vi "Settings - NI 9234.vi"(8 "Error In":errorcluster) -> (0 "Error Out":errorcluster={"status"=TRUE, "code"=-200077, "source"="Property Node DAQmx Channel (arg 2) in DAQmx Create Channel (AI-Temperature-Thermocouple).vi:1->Settings - NI 9211.vi <append>\n<B>Property: </B>AI.Temp.Units\n<B>Requested Value: </B>\n<B>You Can Select: </B>Deg C, Deg F, Kelvins, Deg R, From Custom Scale\n\n<B>Channel Name: </B>Temperature\n\n<B>Task Name: </B>_unnamedTask<E>"}, 3 "Cancelled?":bool)   [LabVIEW 2011]
doc: "This VI will get settings for NI 9211 measurement."
uses:
  SubVIs/Controls/4ch.ctl
  SubVIs/Controls/TransparencyEffectOperations.ctl
  <vilib>/DAQmx/create/channels.llb/DAQmx Create Channel (AI-Acceleration-Accelerometer).vi
  <vilib>/DAQmx/configure/timing.llb/DAQmx Timing (Sample Clock).vi
  Program Files/National Instruments/LabVIEW 2011/resource/objmgr/daqmx.rc
panel:
  in  "Rate":dbl=25600.0
  in  "Nr of Samples":i32=10000
  in  "Sample Mode":i32(ring)=10123 items=["Finite Samples"=10178, "Continuous Samples"=10123, "Hardware Timed Single Point"=12522]
  in  "dB Reference":dbl=1.0
  in  "Sensitivity":dbl=1000.0
  in  "Sensitivity Units":i32(ring)=12509 items=["mVolts/g"=12509, "Volts/g"=12510]
  in  "Unit":i32(ring)=10186 items=["g"=10186, "m/s^2"=12470, "From Custom Scale"=10065]
  in  "Input Terminal Configuration":i32(ring)=12529 items=["default"=-1, "RSE"=10083, "NRSE"=10078, "Differential"=10106, "Pseudodifferential"=12529]
  in  "Excitation Source":i32(ring)=10200 items=["Internal"=10200, "External"=10167, "None"=10230]
  in  "Excitation Value":dbl=0.002
  in  "Channel":T1
  in  "Min":dbl=-5.0
  in  "Max":dbl=5.0
  in  "Header For Measurement File":string="Acceleration 1"
  in  "Cancel Button":bool
  in  "OK Button":bool
  # "NI 9234"
  # "Meas File Settings"
  # "Hardware Settings"
  # "Signal Input Range"
  # "Units"
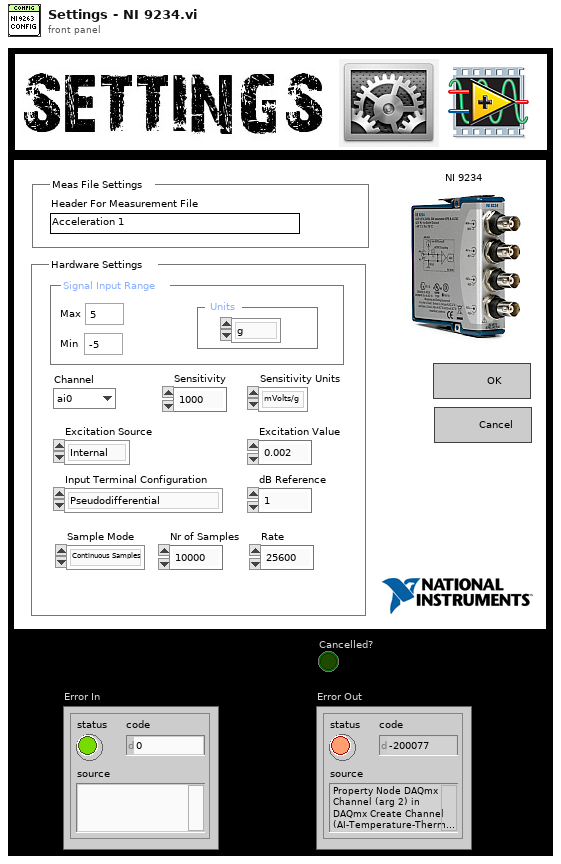
[diagram p1: front panel]
types:
  T1 = typedef "4ch.ctl" = enum16{"ai0", "ai1", "ai2", "ai3"}
  T2 = typedef "TransparencyEffectOperations.ctl" = enum16{"Show", "Hide 80%", "Hide All"}
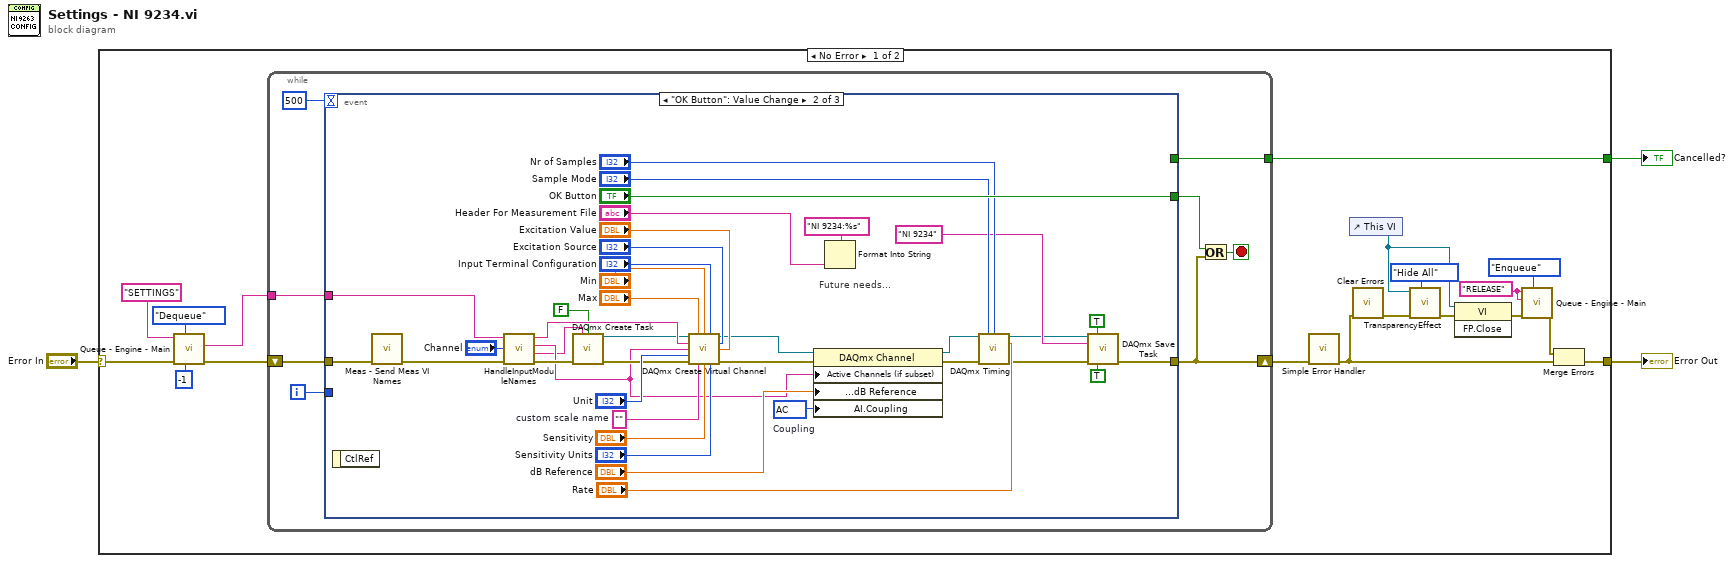
[diagram p0: block diagram]
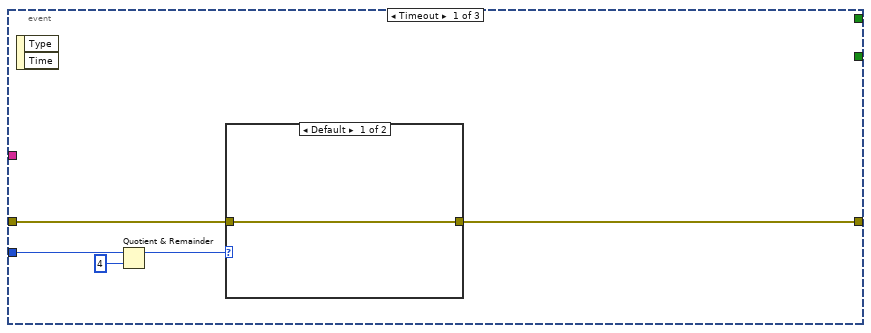
[diagram p2: hidden frame]
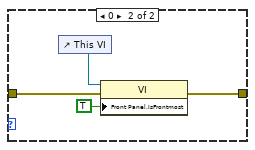
[diagram p3: hidden frame]
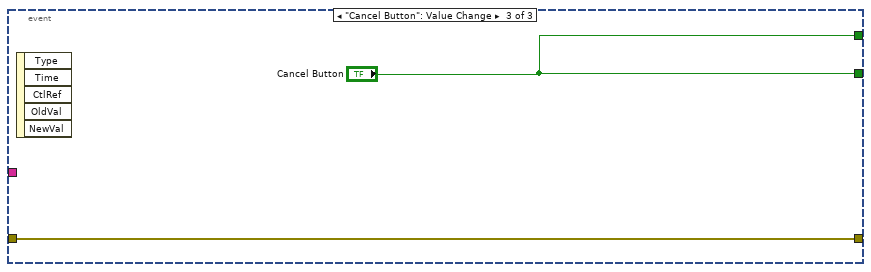
[diagram p4: hidden frame]
diagram:
  n1 = case shown="No Error" "Error In" {
    selector: "Error In" -> [w17 w80]
    tunnel: [w21 _] -> w3
    tunnel: [w4 w80] -> w2
    frame No Error {
      w10 = "RELEASE" ("Queue Data In")
      n2 = call "Queue - Engine - Main.vi"("timeout in ms (-1)"=-1, "Operation"=enum16{"Enqueue", "Dequeue", "Flush", "Release"}."Dequeue", "error in"=w17, "Queue Name In"="SETTINGS") -> ("error out"=w18:errorcluster, "Data Out"=w16:string)  [unwired: 5 in, 1 out]
      n3 = while {
        tunnel: [w29] -> w21
        shift-right: [w24] -> w5
        shift-left: w18 -> [w28]
        tunnel: w16 -> [w25]
        i -> [w26]
        stop <- w22 stop-if-true
        n4 = event shown="[1] \"OK Button\": Value Change" {
          selector: _ -> [_ _ _]
          dyn-events: _ -> [_ _ _]
          timeout: 500 -> [_ _ _]
          tunnel: [_ "OK Button" "Cancel Button"] -> w23
          tunnel: [_ _ "Cancel Button"] -> w29
          tunnel: [w33 w43 w78] -> w24
          tunnel: w28 -> [w34 w47 w78]
          tunnel: w26 -> [w32 _ _]
          tunnel: w25 -> [_ w61 _]
          event Timeout {
            n5 = event-data() -> ()  [unwired: 1 in, 2 out]
            n6 = Quotient & Remainder(x=w32, y=4) -> (x-y*floor(x/y)=w30:i32)  [unwired: 1 out]
            n7 = case shown="Default" w30 {
              tunnel: w34 -> [w35 w38]
              tunnel: [w35 w37] -> w33
              frame Default {
              }
              frame 0 {
                n8 = control-ref of="This VI"() -> (w39:refnum<vi>)
                n9 = property class="VI"(reference=w39, error in=w38, "Front Panel.IsFrontmost"=TRUE ("Front Panel Window:Is Frontmost")) -> (error out=w37:errorcluster)  [unwired: 1 out]
              }
            }
          }
          event "OK Button": Value Change {
            w76 = 10045 items=["AC"=10045, "DC"=10050, "GND"=10066]  # Coupling
            w66 = ""  # custom scale name
            # "Future needs..."
            n10 = event-data() -> ()  [unwired: 1 in, 1 out]
            n11 = call "Meas - Send Meas VI Names.vi"("Error In"=w47) -> ("Error Out"=w46:errorcluster)  [unwired: 10 in]
            n12 = call "HandleInputModuleNames.vi"("Error In"=w46, "Channel"="Channel", "Data In"=w61) -> ("Error Out"=w60:errorcluster, "Meas Name"=w54:string, "Module and CH"=w57:string, "Channel"=w62:string)  [unwired: 5 in]
            n13 = call <vilib>:"DAQmx Create Task.vi"("new task name"=w54, "auto cleanup"=FALSE, "error in"=w60) -> ("task out"=w59:refnum<k21>, "error out"=w63:errorcluster)  [unwired: 2 in, 9 out]
            n14 = call-poly <vilib>:"DAQmx Create Virtual Channel.vi"("task in"=w59, "maximum value"="Max", "minimum value"="Min", "input terminal configuration"="Input Terminal Configuration", "physical channels"=w62, "current excitation source"="Excitation Source", "name to assign"=w57, "current excitation value"="Excitation Value", "units"="Unit", "error in"=w63, "custom scale name"=w66, "sensitivity"="Sensitivity", "sensitivity units"="Sensitivity Units") -> ("task out"=w67:refnum<k21>, "error out"=w74:errorcluster)  [unwired: 1 out]
            n15 = property class="DAQmx Channel"(reference=w67, error in=w74, "Active Channels (if subset)"=w57, "Analog Input:Acceleration:dB Reference"="dB Reference", "AI.Coupling"=w76) -> (reference out=w48:refnum<k21>, error out=w49:errorcluster)
            n16 = Format Into String(format string="NI 9234:%s", "Header For Measurement File") -> ()  [unwired: 2 in, 2 out]
            n17 = call-poly <vilib>:"DAQmx Timing.vi"("task/channels in"=w48, "sample mode"="Sample Mode", "samples per channel"="Nr of Samples", "rate"="Rate", "error in"=w49) -> ("task out"=w40:refnum<k21>, "error out"=w42:errorcluster)  [unwired: 2 in, 7 out]
            n18 = call <vilib>:"DAQmx Save Task.vi"("task/channels in"=w40, "allow interactive editing?"=TRUE, "save as"="NI 9234" ("format string"), "error in"=w42, "overwrite existing task?"=TRUE) -> ("error out"=w43:errorcluster)  [unwired: 9 in, 1 out]
          }
          event "Cancel Button": Value Change {
            n19 = event-data() -> ()  [unwired: 1 in, 5 out]
          }
        }
        n20 = Or(x=w23, y=w24) -> (x .or. y?=w22:bool)
      }
      n21 = call <vilib>:"Simple Error Handler.vi"("error in (no error)"=w5) -> ("error out"=w7:errorcluster)  [unwired: 4 in, 4 out]
      n22 = control-ref of="This VI"() -> (w14:refnum<vi>)
      n23 = call <vilib>:"Clear Errors.vi"("error in (no error)"=w7) -> ("error out"=w6:errorcluster)  [unwired: 6 in]
      n24 = call "TransparencyEffect.vi"("Operation"=TransparencyEffectOperations."Hide All", "error in"=w6, "VI Ref in"=w14) -> ("error out"=w11:errorcluster)  [unwired: 8 in]
      n25 = invoke class="VI" method="FP.Close"(reference=w14, error in=w11) -> (error out=w8:errorcluster)  [unwired: 1 in, 2 out]
      n26 = call "Queue - Engine - Main.vi"("Operation"=enum16{"Enqueue", "Dequeue", "Flush", "Release"}."Enqueue", "error in"=w8, "Queue Data In"=w10, "Queue Name In"=w10) -> ("error out"=w9:errorcluster)  [unwired: 5 in, 2 out]
      n27 = Merge Errors(w9, w7) -> (w4:errorcluster)
    }
    frame Error {
    }
  }
  "Cancelled?" <- w3
  "Error Out" <- w2
